vi "closeCameraManager.vi"(8 "error in (no error)":errorcluster, 11 "CameraManager in":refnum<class "CameraManager.lvclass">) -> (0 "error out":errorcluster, 3 "CameraManager out":refnum<class "CameraManager.lvclass">)   [LabVIEW 2011, in "iManagement.lvlib" / "CameraManager.lvclass"]
uses:
  CameraManager.lvclass
  CameraManager.lvclass/CameraManager.ctl
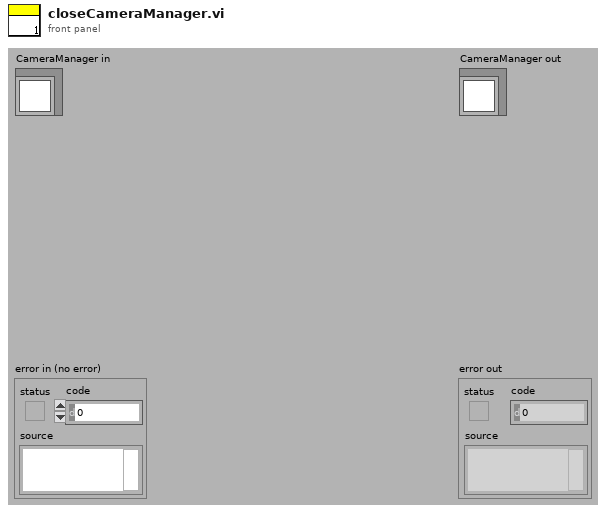
[diagram p1: front panel]
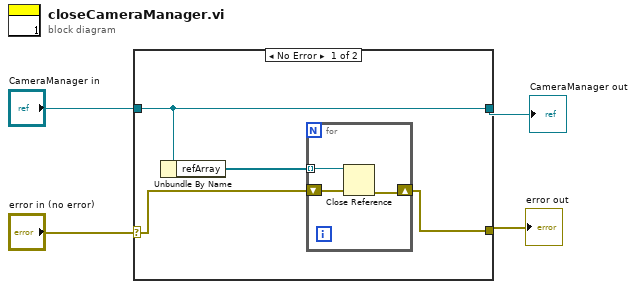
[diagram p0: block diagram]
diagram:
  n1 = case shown="No Error" "error in (no error)" {
    selector: "error in (no error)" -> [w6 w13]
    tunnel: [w5 w13] -> w3
    tunnel: [w8 w12] -> w1
    tunnel: "CameraManager in" -> [w8 w12]
    frame No Error {
      n2 = Unbundle By Name(w8) -> ("refArray"=w7:refnum<vi>[])
      n3 = for {
        tunnel: w7 -> [w11] mode=indexing
        shift-right: [w9] -> w5
        shift-left: w6 -> [w10]
        n4 = Close Reference(reference=w11, error in (no error)=w10) -> (error out=w9:errorcluster)
      }
    }
    frame Error {
    }
  }
  "error out" <- w3
  "CameraManager out" <- w1
